vi "Control - Generic - Rail Pressure Host.vi"() -> ()   [LabVIEW 2015, in "ECS-Host.lvlib"]
uses:
  ECS-Host.lvlib
  <vilib>/addons/Software Calibration Management/XControls/TBL2D.xctl
panel:
  in  "RailP_ManE":bool
  in  "RailP_Man":sgl caption="[bar]"
  out "RailP_Des":sgl caption="[bar]"
  out "RailP_TblOut":sgl caption="[bar]"
  in  "RailP_Tbl":cluster{"X":sgl[], "Y":sgl[], "Z":sgl[][]}(xcontrol)
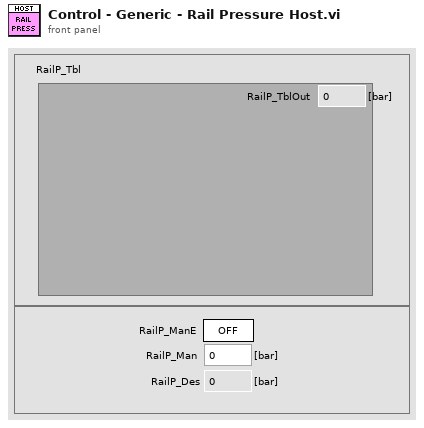
[diagram p1: front panel]
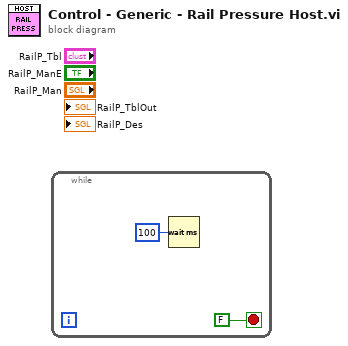
[diagram p0: block diagram]
diagram:
  n1 = while {
    stop <- FALSE stop-if-true
    n2 = Wait (ms)(milliseconds to wait=u32 100) -> ()  [unwired: 1 out]
  }
